vi "模拟输出_连续(多通道).vi"() -> ()   [LabVIEW 2013]
doc: "This example demonstrates how to output a continuous periodic waveform."
uses:
  <userlib>/ArtDAQ/_SubVI/ArtDAQ_CreateAOVoltageChan.vi
  <userlib>/ArtDAQ/_SubVI/ArtDAQ_CfgSampClkTiming.vi
  <userlib>/ArtDAQ/_SubVI/ArtDAQ_Write Analog DBL NChan NSamp.vi
  <userlib>/ArtDAQ/_SubVI/ArtDAQ_CfgDigEdgeStartTrig.vi
  <vilib>/Analysis/NI_AALBase.lvlib
panel:
  in  "周期点数":dbl=1000.0 format="%#_13g"
  in  "幅值(V)":dbl=3.0 format="%#_13g"
  in  "?":enum32{"无触发 ", "数字边沿触发"}(tab)
  in  "触发源":string="/Dev1/PFI1"
  in  "触发边沿":i32(ring)=10280 items=["上升"=10280, "下降"=10171]
  in  "Stop":bool
  out "Waveform":dbl[][](graph)
  in  "采样速率":dbl=1000.0
  in  "每通道输出点数":i32=4000
  in  "最大值(V)":dbl=10.0
  in  "最小值(V)":dbl=-10.0
  in  "物理通道":string(combo)="Dev1/ao0:1"
  out "错误输出":errorcluster
  # "通道属性"
  # "定时"
  # "波形"
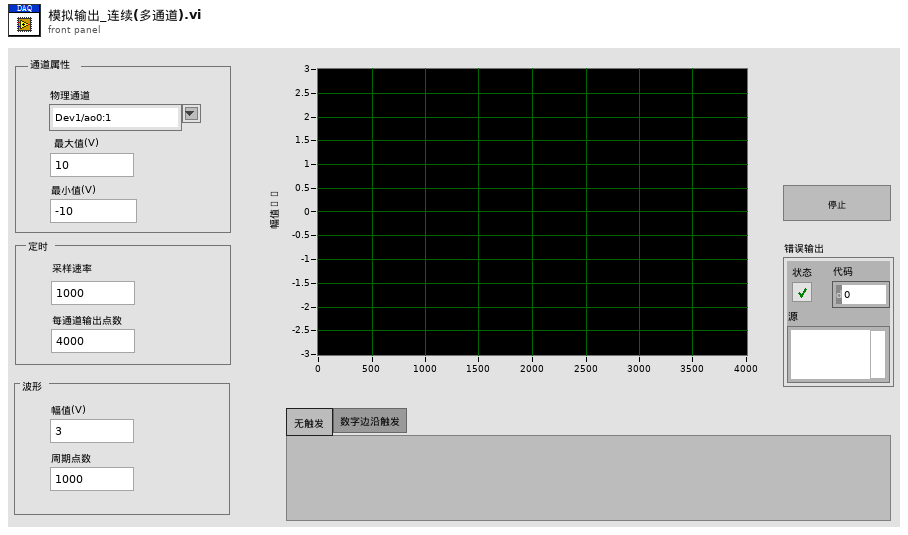
[diagram p1: front panel]
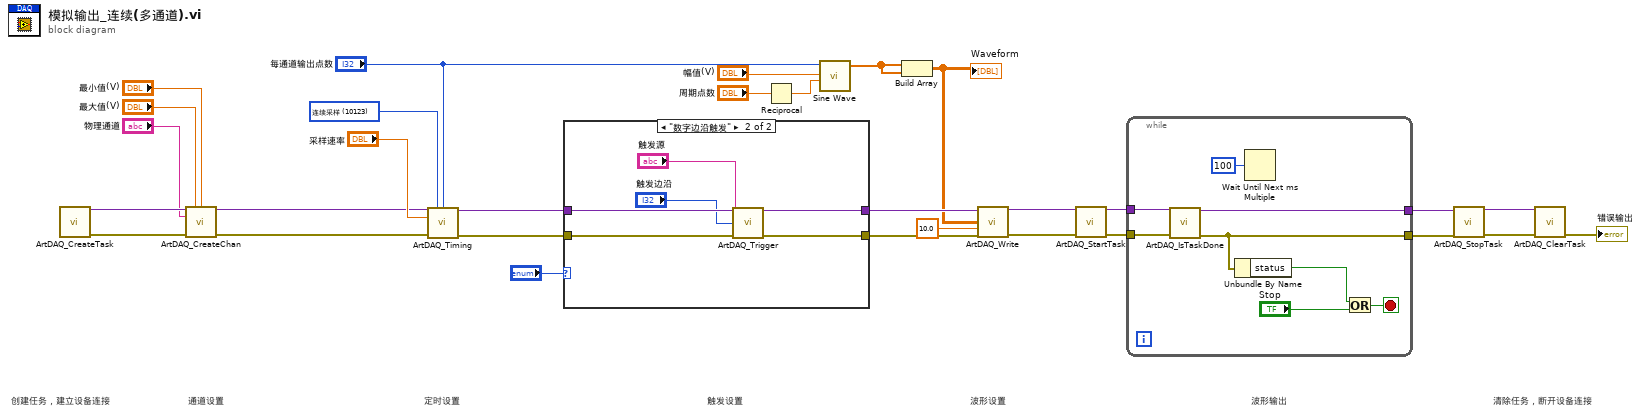
[diagram p0: block diagram]
diagram:
  w19 = 10123 items=["有限点采样"=10178, "连续采样"=10123] ("SampleMode")
  # "清除任务，断开设备连接"
  # "波形输出"
  # "波形设置"
  # "触发设置"
  # "定时设置"
  # "通道设置"
  # "创建任务，建立设备连接"
  n1 = call <userlib>:"ArtDAQ_CreateTask.vi"() -> ("任务句柄"=w30:variant, "错误输出"=w29:errorcluster)  [unwired: 14 in]
  n2 = call-poly <userlib>:"ArtDAQ_CreateChan.vi"("任务句柄"=w30, "最大值"="最大值(V)", "最小值"="最小值(V)", "物理通道"="物理通道", "错误输入"=w29) -> ("任务句柄"=w11:variant, "错误输出"=w21:errorcluster)  [unwired: 9 in]
  n3 = call-poly <userlib>:"ArtDAQ_Timing.vi"("任务句柄"=w11, "采样模式"=w19, "每通道采样数"="每通道输出点数", "采样率"="采样速率", "错误输入"=w21) -> ("任务句柄"=w10:variant, "错误输出"=w8:errorcluster)  [unwired: 9 in]
  n4 = case shown="\"数字边沿触发\"" "?" {
    tunnel: w10 -> [w32 w38]
    tunnel: [w32 w37] -> w9
    tunnel: w8 -> [w31 w35]
    tunnel: [w31 w36] -> w7
    frame "无触发 ", Default {
    }
    frame "数字边沿触发" {
      n5 = call-poly <userlib>:"ArtDAQ_Trigger.vi"("任务句柄"=w38, "触发源"="触发源", "边沿"="触发边沿", "错误输入"=w35) -> ("任务句柄"=w37:variant, "错误输出"=w36:errorcluster)  [unwired: 10 in]
    }
  }
  n6 = Reciprocal(x="周期点数") -> (1/x=w12:dbl)
  n7 = call <vilib>:"Sine Wave.vi"("samples"="每通道输出点数", "amplitude"="幅值(V)", "frequency"=w12) -> ("sine wave"=w3:dbl[])  [unwired: 2 in, 2 out]
  n8 = Build Array(w3, w3) -> (w2:dbl[][])
  "Waveform" <- w2
  n9 = call-poly <userlib>:"ArtDAQ_Write.vi"("任务句柄"=w9, "数据"=w2, "超时s"=10.0 ("Timeout"), "错误输入"=w7) -> ("任务句柄"=w17:variant, "错误输出"=w18:errorcluster)  [unwired: 9 in, 1 out]
  n10 = call <userlib>:"ArtDAQ_StartTask.vi"("任务句柄"=w17, "错误输入"=w18) -> ("任务句柄"=w16:variant, "错误输出"=w15:errorcluster)  [unwired: 12 in]
  n11 = while {
    tunnel: w16 -> [w46]
    tunnel: w15 -> [w40]
    tunnel: [w45] -> w14
    tunnel: [w39] -> w13
    stop <- w42 stop-if-true
    n12 = call <userlib>:"ArtDAQ_IsTaskDone.vi"("任务句柄"=w46, "错误输入"=w40) -> ("任务句柄"=w45:variant, "错误输出"=w39:errorcluster)  [unwired: 11 in, 1 out]
    n13 = Unbundle By Name(w39) -> ("status"=w43:bool)
    n14 = Wait Until Next ms Multiple(millisecond multiple=u32 100 ("毫秒倍数")) -> ()  [unwired: 1 out]
    n15 = Or(x=w43, y="Stop") -> (x .or. y?=w42:bool)
  }
  n16 = call <userlib>:"ArtDAQ_StopTask.vi"("任务句柄"=w14, "错误输入"=w13) -> ("任务句柄"=w28:variant, "错误输出"=w27:errorcluster)  [unwired: 12 in]
  n17 = call <userlib>:"ArtDAQ_ClearTask.vi"("任务句柄"=w28, "错误输入"=w27) -> ("错误输出"=→"错误输出":errorcluster)  [unwired: 13 in]
